vi "RTS Calculate Door Openings.vi"(8 "Error In":errorcluster, 9 "Standard Tests 1-1":T1, 10 "Current Index":u32, 11 "Input":T2[](array[typedef]) {"Start Time" format="%<%X\n%x>T"; "End Time" format="%<%X\n%x>T"}) -> (0 "Error Out":errorcluster, 3 "Output":T2[](array[typedef]) {"Start Time" format="%<%X\n%x>T"; "End Time" format="%<%X\n%x>T"})   [LabVIEW 2016]
uses:
  Type Definitions/RTS Door Ops Client.ctl
  Type Definitions/RTS Door Opening Schedule.ctl
  Type Definitions/RTS Door Ops Sequence.ctl
  Type Definitions/RTS Standard Door Opening Test.ctl
panel:
  # "Chamber Conditions:"
  # "Chamber Conditions:"
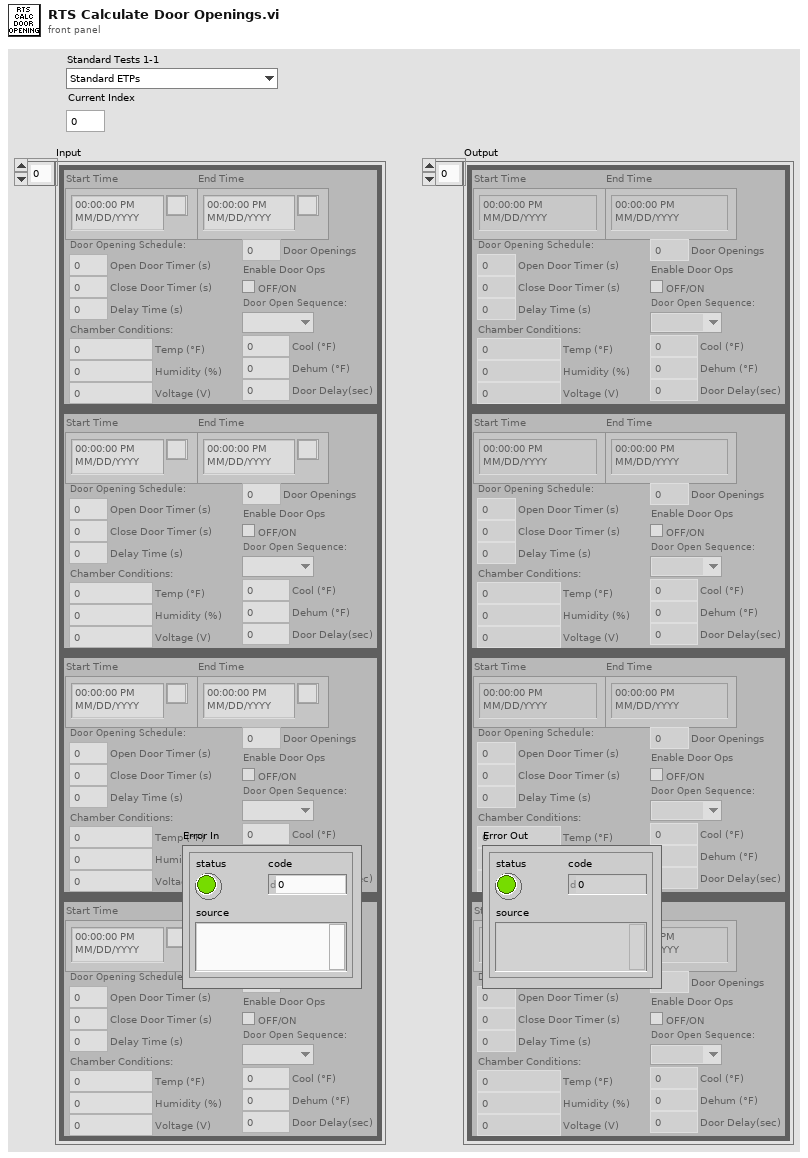
[diagram p1: front panel]
types:
  T1 = typedef "RTS Standard Door Opening Test.ctl" = enum16{"Standard ETPs", "511-B113 EHUT", "511-B110 HUT", "512-C410 SLAT", "511-B111 Internal Moisture", "511-C401 Moisture Accumulation", "511-B100 No Door Opening (NDO)", "511-B304 ISO Energy Consumption", "Custom Test", "Cancel Test"}
  T2 = typedef "RTS Door Ops Client.ctl" = cluster{"End Time":timestamp, "Start Time":timestamp, "Door Opening Schedule:":T3, "Enable Door Ops":bool, "Door Openings":u32, "Temp (°F)":dbl, "Humidity (%)":dbl, "Voltage (V)":dbl, "Door Open Sequence:":T4, "Door Delay(sec)":dbl, "Dehum (°F)":dbl, "Cool (°F)":dbl}
  T3 = typedef "RTS Door Opening Schedule.ctl" = cluster{"Open Door Timer (s)":dbl, "Delay Time (s)":dbl, "Close Door Timer (s)":dbl}
  T4 = typedef "RTS Door Ops Sequence.ctl" = enum16{"", "1st", "2nd", "3rd"}
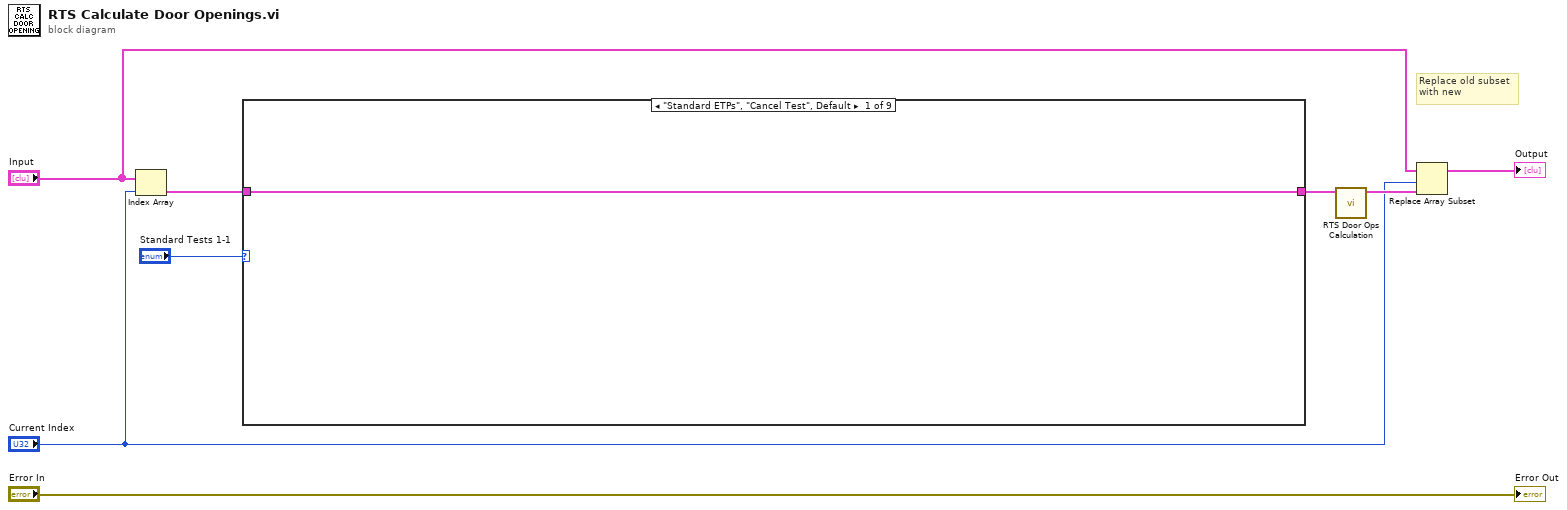
[diagram p0: block diagram]
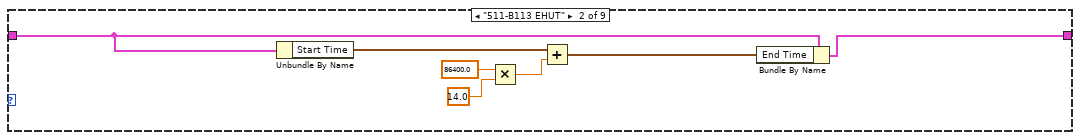
[diagram p2: hidden frame]
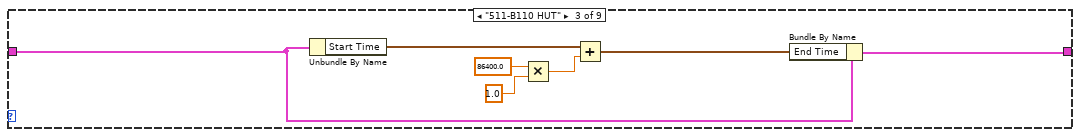
[diagram p3: hidden frame]
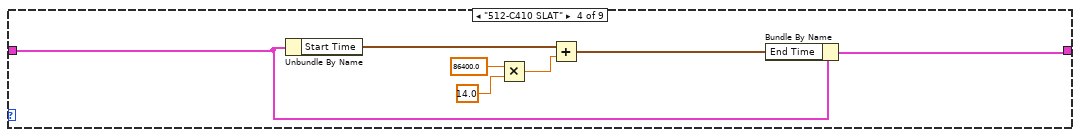
[diagram p4: hidden frame]
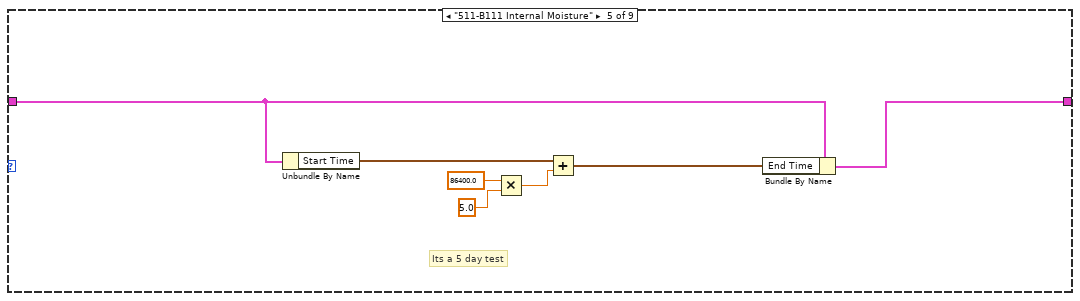
[diagram p5: hidden frame]
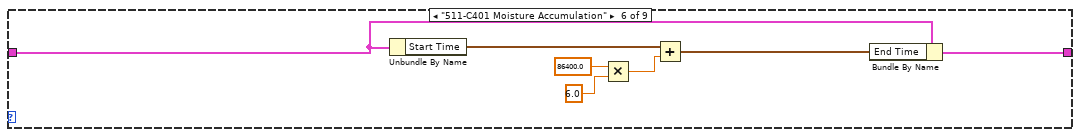
[diagram p6: hidden frame]
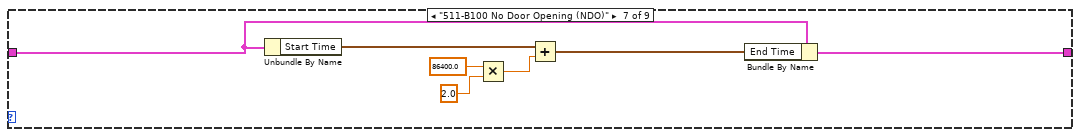
[diagram p7: hidden frame]
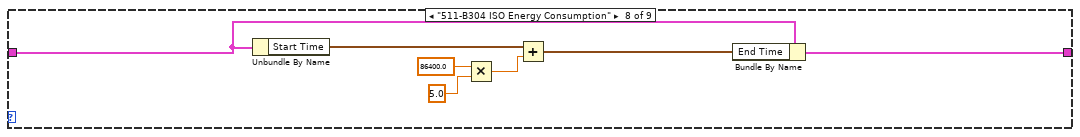
[diagram p8: hidden frame]
diagram:
  # "Replace old subset\nwith new"
  n1 = Index Array(array="Input", index="Current Index") -> (element=w2:T2)
  n2 = case shown="\"Standard ETPs\", \"Cancel Test\", Default" "Standard Tests 1-1" {
    tunnel: w2 -> [w9 w10 w17 w25 w34 w38 w46 w53 w59]
    tunnel: [w9 w11 w18 w24 w33 w39 w45 w52 w59] -> w1
    frame "Standard ETPs", "Cancel Test", Default {
    }
    frame "511-B113 EHUT" {
      n3 = Unbundle By Name(w10) -> ("Start Time"=w14:timestamp)
      n4 = Multiply(x=86400.0, y=14.0) -> (x*y=w12:dbl)
      n5 = Add(x=w14, y=w12) -> (x+y=w13:timestamp)
      n6 = Bundle By Name(cluster=w10, "End Time"=w13) -> (w11:T2)
    }
    frame "511-B110 HUT" {
      n7 = Unbundle By Name(w17) -> ("Start Time"=w21:timestamp)
      n8 = Multiply(x=86400.0, y=1.0) -> (x*y=w19:dbl)
      n9 = Add(x=w21, y=w19) -> (x+y=w20:timestamp)
      n10 = Bundle By Name(cluster=w17, "End Time"=w20) -> (w18:T2)
    }
    frame "512-C410 SLAT" {
      n11 = Unbundle By Name(w25) -> ("Start Time"=w28:timestamp)
      n12 = Multiply(x=86400.0, y=14.0) -> (x*y=w26:dbl)
      n13 = Add(x=w28, y=w26) -> (x+y=w27:timestamp)
      n14 = Bundle By Name(cluster=w25, "End Time"=w27) -> (w24:T2)
    }
    frame "511-B111 Internal Moisture" {
      # "Its a 5 day test"
      n15 = Unbundle By Name(w34) -> ("Start Time"=w35:timestamp)
      n16 = Multiply(x=86400.0, y=5.0) -> (x*y=w31:dbl)
      n17 = Add(x=w35, y=w31) -> (x+y=w32:timestamp)
      n18 = Bundle By Name(cluster=w34, "End Time"=w32) -> (w33:T2)
    }
    frame "511-C401 Moisture Accumulation" {
      n19 = Unbundle By Name(w38) -> ("Start Time"=w42:timestamp)
      n20 = Multiply(x=86400.0, y=6.0) -> (x*y=w40:dbl)
      n21 = Add(x=w42, y=w40) -> (x+y=w41:timestamp)
      n22 = Bundle By Name(cluster=w38, "End Time"=w41) -> (w39:T2)
    }
    frame "511-B100 No Door Opening (NDO)" {
      n23 = Unbundle By Name(w46) -> ("Start Time"=w49:timestamp)
      n24 = Multiply(x=86400.0, y=2.0) -> (x*y=w47:dbl)
      n25 = Add(x=w49, y=w47) -> (x+y=w48:timestamp)
      n26 = Bundle By Name(cluster=w46, "End Time"=w48) -> (w45:T2)
    }
    frame "511-B304 ISO Energy Consumption" {
      n27 = Unbundle By Name(w53) -> ("Start Time"=w56:timestamp)
      n28 = Multiply(x=86400.0, y=5.0) -> (x*y=w54:dbl)
      n29 = Add(x=w56, y=w54) -> (x+y=w55:timestamp)
      n30 = Bundle By Name(cluster=w53, "End Time"=w55) -> (w52:T2)
    }
    frame "Custom Test" {
    }
  }
  n31 = call "RTS Door Ops Calculation.vi"("Chamber 1-1 in"=w1) -> ("Chamber 1-1 out"=w7:T2)  [unwired: 9 in, 1 out]
  n32 = Replace Array Subset(array="Input", new element=w7, index="Current Index") -> (→"Output":T2[])
  "Error Out" <- "Error In"
